vi "FlatToRichrfcontrol_USBResponse.vi"(5 "OutputClusterType":T1, 11 "InputCluster":T2) -> (3 "OutputCluster":T1)   [LabVIEW 2024, in "FlexSDR_gRPC_client.lvlib"]
uses:
  FlexSDR_gRPC_client.lvlib
  rfcontrol_USBResponse_Flat.ctl
  rfcontrol_USBResponse.ctl
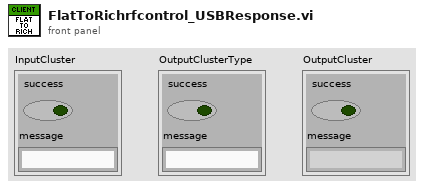
[diagram p1: front panel]
types:
  T1 = typedef "FlexSDR_gRPC_client.lvlib/rfcontrol_USBResponse.ctl" = cluster{"success":bool, "message":string}
  T2 = typedef "FlexSDR_gRPC_client.lvlib/rfcontrol_USBResponse_Flat.ctl" = cluster{"success":bool, "message":string}
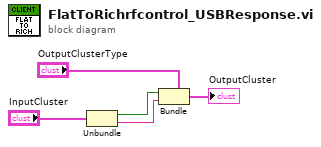
[diagram p0: block diagram]
diagram:
  n1 = Unbundle "Unbundle"("InputCluster") -> ("success"=w2:bool, "message"=w1:string)
  n2 = Bundle "Bundle"(cluster="OutputClusterType", "success"=w2, "message"=w1) -> (→"OutputCluster":T1)
